vi "Query Gate mode.vi"(8 "error in (no error)":errorcluster, 10 "i (0)":T2, 11 "VISA resource name":refnum<visa-resource-name>) -> (0 "error out":errorcluster, 2 "Gate mode":T1, 3 "VISA resource name out":refnum<visa-resource-name>)   [LabVIEW 2015, in "SR400.lvlib"]
doc: "GM i { ,j }\nThe GM command sets and reads the gate modes. i\n= 0 or 1 designates A gate or B gate and is\nrequired. If j is included, the selected gate is set to\nCW, j=0, or FIXED, j=1, or SCAN, j=2. If j is\nabsent, the mode of gate i is returned. The mode\nmay be changed during a scan. If it is changed to\nSCAN, the delay begins scanning from the start\nposition on the next count period. If it is changed\nto FIXED, the delay returns to the start position\nimmediately. If it is changed to CW, the gate\nimmediately changes to continuously on."
uses:
  SR400.lvlib
  Typedefs/Gate.ctl
  Typedefs/Gate Mode.ctl
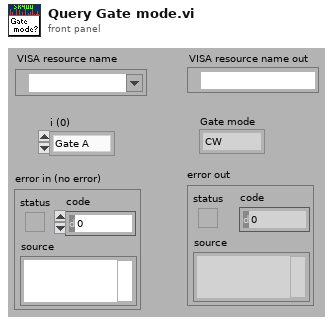
[diagram p1: front panel]
types:
  T1 = typedef "SR400.lvlib/Gate Mode.ctl" = enum16{"CW", "Fixed", "Scan"}
  T2 = typedef "SR400.lvlib/Gate.ctl" = enum16{"Gate A", "Gate B"}
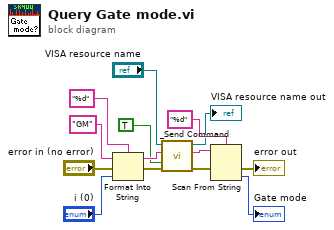
[diagram p0: block diagram]
diagram:
  n1 = Format Into String(format string="%d", initial string="GM" ("command"), error in="error in (no error)", "i (0)") -> (resulting string=w7:string, error out=w6:errorcluster)
  n2 = call "_Send Command.vi"("error in (no error)"=w6, "Query? (F)"=TRUE, "Command"=w7, "VISA resource name"="VISA resource name") -> ("error out"=w3:errorcluster, "Response"=w4:string, "VISA resource name out"=→"VISA resource name out":refnum<visa-resource-name>)  [unwired: 5 out]
  n3 = Scan From String(format string="%d", input string=w4, error in=w3) -> (error out=→"error out":errorcluster, output 1=→"Gate mode":T1)  [unwired: 1 in, 3 out]
